vi "preset diagnostics GUI.vi"(11 "preset diagnostics":T1) -> ()   [LabVIEW 2018]
uses:
  preset diagnostics.ctl
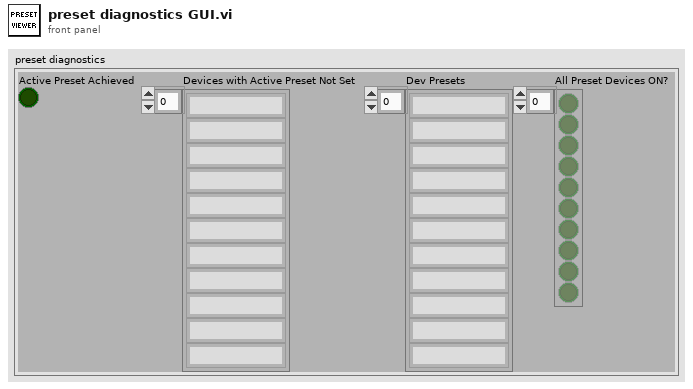
[diagram p1: front panel]
types:
  T1 = typedef "preset diagnostics.ctl" = cluster{"Active Preset Achieved":bool, "Devices with Active Preset Not Set":string[], "Dev Presets":string[], "All Preset Devices ON?":bool[]}
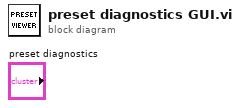
[diagram p0: block diagram]
diagram:
